vi "OPC_Hex_String.vi"(4 "HexInput":u32) -> (0 "number":i32, 2 "Str Number":string)   [LabVIEW 2017]
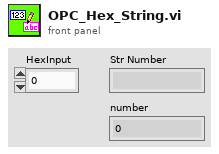
[diagram p1: front panel]
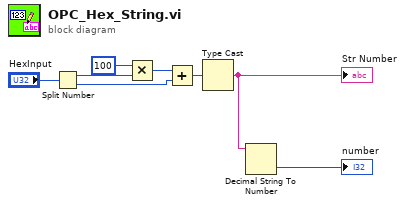
[diagram p0: block diagram]
diagram:
  n1 = Split Number(x="HexInput") -> (hi(x)=w8:u16, lo(x)=w5:u16)
  n2 = Multiply(x=u16 100, y=w8) -> (x*y=w6:u16)
  n3 = Add(x=w6, y=w5) -> (x+y=w4:u16)
  n4 = Type Cast(x=w4) -> (*(type *) &x=w2:string)  [unwired: 1 in]
  "Str Number" <- w2
  n5 = Decimal String To Number(string=w2) -> (number=→"number":i32)  [unwired: 2 in, 1 out]
